vi "Добавить точку на рисунок (SubVI).vi"(0 "in picture":picture, 2 "id мишени вх":u16 step=1, 4 "цвет":u32(colorbox), 5 "error in":errorcluster, 8 "dot х":u16 step=1, 9 "dot y":u16 step=1) -> (14 "error out":errorcluster, 16 "id мишени вых":u16 step=1, 19 "out picture":picture)   [LabVIEW 2015]
panel:
  in  "Style":T1(ring)
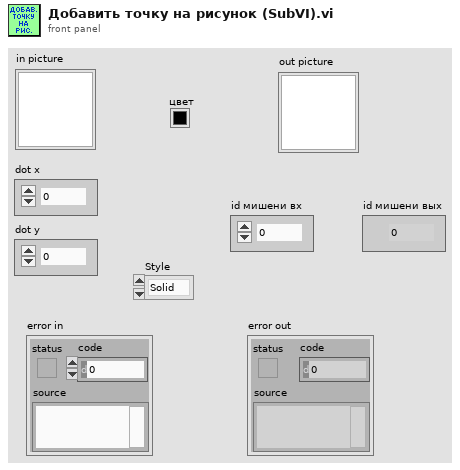
[diagram p1: front panel]
types:
  T1 = enum32{"Solid", "Dash", "Dot", "DashDot", "DashDotDot"}
  T2 = cluster{"y":u16, "Style":enum32{"Solid", "Dash", "Dot", "DashDot", "DashDotDot"}}
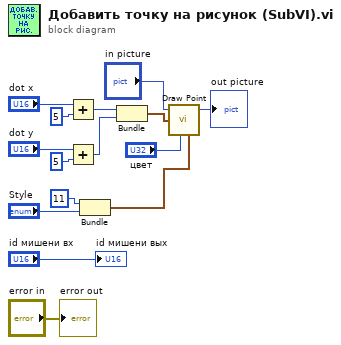
[diagram p0: block diagram]
diagram:
  n1 = Add(x="dot х", y=u16 5) -> (x+y=w5:u16)
  n2 = Add(x="dot y", y=u16 5) -> (x+y=w6:u16)
  n3 = Bundle("y"=u16 11, "Style"="Style") -> (w14:T2)  [unwired: 1 in]
  n4 = Bundle(w5, w6) -> (w12:cluster{u16, u16})  [unwired: 1 in]
  n5 = call <vilib>:"Draw Point.vi"("picture"="in picture", "point(x,y)"=w12, "color(black)"="цвет", "pen"=w14) -> ("new picture"=→"out picture":picture)  [unwired: 5 in]
  "error out" <- "error in"
  "id мишени вых" <- "id мишени вх"
